vi "MIMO Check.vi"(0 "MIMO State-Space":T1 {"D" format="%.2f"; "C" format="%.2f"; "B" format="%.2f"; "A" format="%.2f"}, 1 "Input Points":dbl[](array[numeric]) format="%.2f") -> (2 "nx":u32, 3 "nu":u32, 4 "ny":u32, 5 "error":i32)   [LabVIEW 2017, in "NI_AdvCtrl_continuous linear.lvlib"]
doc: "LabVIEW no longer supports this VI. You can obtain similar functionality by installing the LabVIEW Simulation Module."
uses:
  <vilib>/addons/control/advanced/NI_AdvCtrl_continuous linear.lvlib
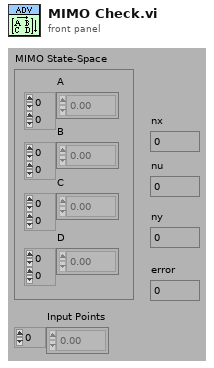
[diagram p1: front panel]
types:
  T1 = cluster{"A":dbl[][], "B":dbl[][], "C":dbl[][], "D":dbl[][]}
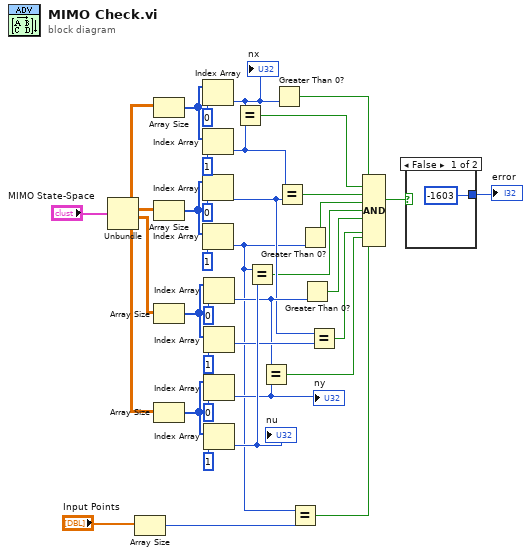
[diagram p0: block diagram]
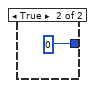
[diagram p2: hidden frame]
diagram:
  n1 = Unbundle("MIMO State-Space") -> ("A"=w31:dbl[][], "B"=w26:dbl[][], "C"=w30:dbl[][], "D"=w29:dbl[][])
  n2 = Array Size(array="Input Points") -> (size(s)=w2:i32)
  n3 = Array Size(array=w31) -> (size(s)=w32:i32[])
  n4 = Array Size(array=w26) -> (size(s)=w19:i32[])
  n5 = Array Size(array=w30) -> (size(s)=w18:i32[])
  n6 = Array Size(array=w29) -> (size(s)=w17:i32[])
  n7 = Index Array(array=w32, index=0) -> (element=w14:i32)
  "nx" <- w14
  n8 = Index Array(array=w32, index=1) -> (element=w13:i32)
  n9 = Index Array(array=w19, index=0) -> (element=w9:i32)
  n10 = Index Array(array=w19, index=1) -> (element=w3:i32)
  n11 = Index Array(array=w18, index=0) -> (element=w10:i32)
  n12 = Index Array(array=w18, index=1) -> (element=w11:i32)
  n13 = Index Array(array=w17, index=0) -> (element=w8:i32)
  "ny" <- w8
  n14 = Index Array(array=w17, index=1) -> (element=w12:i32)
  "nu" <- w12
  n15 = Equal?(x=w14, y=w13) -> (x = y?=w35:bool)
  n16 = Equal?(x=w3, y=w12) -> (x = y?=w7:bool)
  n17 = Equal?(x=w10, y=w8) -> (x = y?=w15:bool)
  n18 = Greater Than 0?(x=w14) -> (x > 0?=w33:bool)
  n19 = Equal?(x=w13, y=w9) -> (x = y?=w34:bool)
  n20 = Equal?(x=w3, y=w2) -> (x = y?=w1:bool)
  n21 = Greater Than 0?(x=w3) -> (x > 0?=w16:bool)
  n22 = Greater Than 0?(x=w10) -> (x > 0?=w5:bool)
  n23 = Equal?(x=w9, y=w11) -> (x = y?=w6:bool)
  n24 = Compound Arithmetic op=AND(w33, w35, w34, w16, w7, w5, w6, w15, w1) -> (w28:bool)
  n25 = case shown="False" w28 {
    tunnel: [-1603 0] -> w27
    frame False {
    }
    frame True {
    }
  }
  "error" <- w27
